vi "Emergency Islanded.vi"(8 "error in (no error)":errorcluster, 11 "SCADA in":refnum<class "SCADA.lvclass">) -> (0 "error out":errorcluster, 3 "SCADA out":refnum<class "SCADA.lvclass">)   [LabVIEW 2015, in "SCADA Core.lvlib" / "SCADA.lvclass"]
uses:
  SCADA.lvclass
  Controls/Grid Mode.ctl
  <vilib>/ActorFramework/Actor/Actor.lvclass/Actor.ctl
  SCADA.lvclass/SCADA.ctl
  <vilib>/ActorFramework/Actor/Actor.lvclass
  SCADA Abstract Messages/Emergency Status Msg/Emergency Status Msg.lvclass
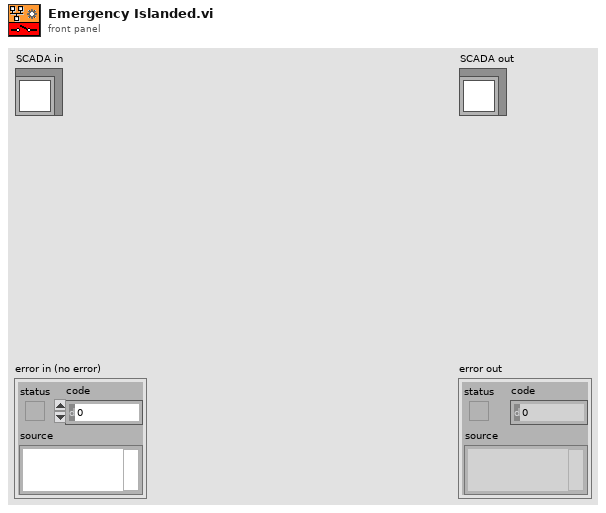
[diagram p1: front panel]
types:
  T1 = typedef "SCADA Core.lvlib/SCADA.lvclass/Grid Mode.ctl" = enum16{"Off", "Grid Connected", "Islanded", "Synchronizing"}
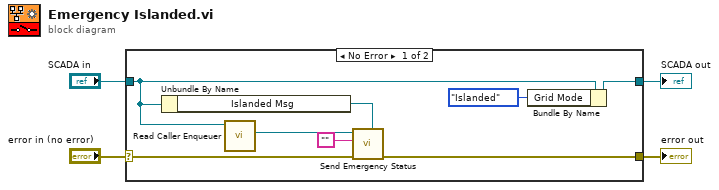
[diagram p0: block diagram]
diagram:
  n1 = case shown="No Error" "error in (no error)" {
    selector: "error in (no error)" -> [w9 w14]
    tunnel: [w8 w14] -> w3
    tunnel: [w6 w13] -> w1
    tunnel: "SCADA in" -> [w7 w13]
    frame No Error {
      n2 = Unbundle By Name(w7) -> ("Islanded Msg"=w12:refnum<class "Emergency Status Msg.lvclass">)
      n3 = call <vilib>:"Read Caller Enqueuer.vi"("Actor"=w7) -> ("Caller Enqueuer"=w11:refnum<class "Message Enqueuer.lvclass">)  [unwired: 10 in]
      n4 = call "Send Emergency Status.vi"("Emergency Status Msg"=w12, "error in (no error)"=w9, "content"="", "Message Enqueuer in"=w11) -> ("error out"=w8:errorcluster)  [unwired: 6 in, 1 out]
      n5 = Bundle By Name(cluster=w7, "Grid Mode"=Grid_Mode."Islanded") -> (w6:refnum<class "SCADA.lvclass">)
    }
    frame Error {
    }
  }
  "error out" <- w3
  "SCADA out" <- w1
